vi "presention_showoff.vi"() -> ()   [LabVIEW 2012]
uses:
  <vilib>/NXT/Subs/LVHSConnector.ctl
  <vilib>/NXT/Subs/MotorOutput.ctl
  <vilib>/NXT/Block Support/NXT_InputPort.ctl
  <vilib>/NXT/Dual Mode Library/Motors/MotorOn.vi
  <vilib>/NXT/Dual Mode Library/Motors/MotorReverse.vi
  <vilib>/NXT/Dual Mode Library/Motors/MotorBrake.vi
  <vilib>/NXT/Dual Mode Library/Display/clearDisplay.vi
  <vilib>/NXT/Dual Mode Library/Waits/Wait_Num(msec).vi
  <vilib>/NXT/Dual Mode Library/Display/drawLine.vi
  <vilib>/NXT/Dual Mode Library/Display/drawNumber.vi
  <vilib>/NXT/Dual Mode Library/Display/drawCircle.vi
  <vilib>/NXT/Dual Mode Library/Waits/Wait_Num.vi
  <vilib>/NXT/Dual Mode Library/prims/addArrayElements_int.vi
  <vilib>/NXT/Dual Mode Library/prims/rotateArray/rotateArray_int.vi
  <vilib>/NXT/Dual Mode Library/Display/drawText.vi
  <vilib>/NXT/Dual Mode Library/Sound/Tone.vi
panel:
  in  "array length 2":i32
  in  "length around index 2":i32
  in  "index 2":i32
  in  "Array 7":i16[](array[numeric])
  out "Array 6":i32[](array[numeric])
  in  "clear (T/F) 4":bool
  in  "array 5":i32[](array[numeric])
  out "NXT 14":T1={"Hardware"="NXT", "Flattened String"=""}
  in  "NXT 13":T1={"Hardware"="NXT", "Flattened String"=""}
  in  "clear (T/F) 3":bool
  in  "array 4":i32[](array[numeric])
  out "NXT 12":T1={"Hardware"="NXT", "Flattened String"=""}
  in  "NXT 11":T1={"Hardware"="NXT", "Flattened String"=""}
  in  "clear (T/F) 2":bool
  in  "array 3":i32[](array[numeric])
  out "NXT 10":T1={"Hardware"="NXT", "Flattened String"=""}
  in  "NXT 9":T1={"Hardware"="NXT", "Flattened String"=""}
  out "Array 5":i16[](array[numeric])
  in  "array 2":i16[](array[numeric])
  out "Array 4":i32[](array[numeric])
  in  "Array 3":i16[](array[numeric])
  in  "clear (T/F)":bool
  in  "array":i32[](array[numeric])
  out "NXT 8":T1={"Hardware"="NXT", "Flattened String"=""}
  in  "NXT 7":T1={"Hardware"="NXT", "Flattened String"=""}
  out "debug array":i32[](array[numeric])
  in  "Array":i16[](array[numeric])
  out "Array 2":i32[](array[numeric])
  out "stuck":bool
  out "NXT 6":T1 caption="NXT"
  in  "min distance":i32=50
  in  "power 2":i32=50
  in  "NXT 5":T1
  in  "power":u16=75
  in  "degrees to  rotate":dbl
  in  "right(T)/left(F) 2":bool
  in  "NXT 4":T1={"Hardware"="NXT", "Flattened String"=""}
  out "NXT 3":T1={"Hardware"="NXT", "Flattened String"=""}
  out "NXT 2":T1={"Hardware"="NXT", "Flattened String"=""}
  out "right(T)/left(F)":bool
  out "angle":dbl
  in  "NXT":T1={"Hardware"="NXT", "Flattened String"=""}
types:
  T1 = typedef "LVHSConnector.ctl" = cluster{"Hardware":string, "Flattened String":string}
  T2 = cluster{"Origin X":i16, "Origin Y":i16, "Radius":u8}
  T3 = typedef "MotorOutput.ctl" = u8
  T4 = typedef "NXT_InputPort.ctl" = u8
  T5 = cluster{"x-y*floor(x/y)":i32, "Start X":i16, "x-y*floor(x/y)":i32, i16}
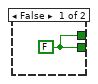
[diagram p2: hidden frame]
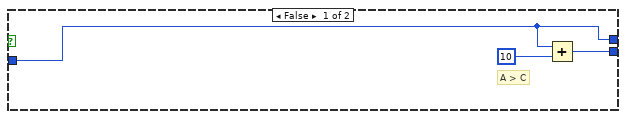
[diagram p3: hidden frame]
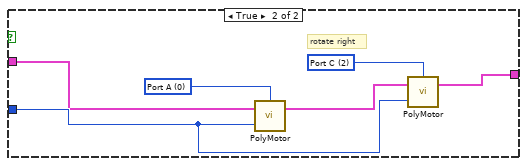
[diagram p5: hidden frame]
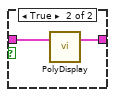
[diagram p7: hidden frame]
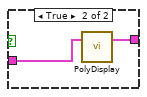
[diagram p12: hidden frame]
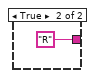
[diagram p14: hidden frame]
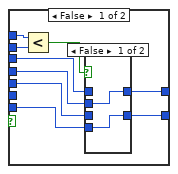
[diagram p17: hidden frame]
diagram:
  n1 = while {
    stop <- FALSE stop-if-true
    w7 = 0
    w10 = T3 5 items=["Port A"=0, "Port B"=1, "Port C"=2, "Ports A & B"=4, "Ports A & C"=5, "Ports B & C"=6, "All Ports"=3] ("Output Port (All Ports)")
    w8 = T3 5 items=["Port A"=0, "Port B"=1, "Port C"=2, "Ports A & B"=4, "Ports A & C"=5, "Ports B & C"=6, "All Ports"=3] ("Output Port (All Ports)")
    w14 = T3 5 items=["Port A"=0, "Port B"=1, "Port C"=2, "Ports A & B"=4, "Ports A & C"=5, "Ports B & C"=6, "All Ports"=3] ("Port (All Ports)")
    w22 = T3 5 items=["Port A"=0, "Port B"=1, "Port C"=2, "Ports A & B"=4, "Ports A & C"=5, "Ports B & C"=6, "All Ports"=3] ("Port (All Ports)")
    w46 = T3 5 items=["Port A"=0, "Port B"=1, "Port C"=2, "Ports A & B"=4, "Ports A & C"=5, "Ports B & C"=6, "All Ports"=3] ("Port (All Ports)")
    w52 = T3 5 items=["Port A"=0, "Port B"=1, "Port C"=2, "Ports A & B"=4, "Ports A & C"=5, "Ports B & C"=6, "All Ports"=3] ("Port (All Ports)")
    w56 = T3 2 items=["Port A"=0, "Port B"=1, "Port C"=2, "Ports A & B"=4, "Ports A & C"=5, "Ports B & C"=6, "as"=3] ("Output Port (All Ports)")
    w54 = T3 0 items=["Port A"=0, "Port B"=1, "Port C"=2, "Ports A & B"=4, "Ports A & C"=5, "Ports B & C"=6, "as"=3] ("Output Port (All Ports)")
    w69 = i16 -1 ("Start X")
    w42 = TRUE
    w51 = 35 ("Power (75)")
    w91 = T3 5 items=["Port A"=0, "Port B"=1, "Port C"=2, "Ports A & B"=4, "Ports A & C"=5, "Ports B & C"=6, "All Ports"=3] ("Port (All Ports)")
    # "Drive forward in a stright line.\nStop if:\n distance to wall is less then X.\n one of the wheels stops rotating"
    # "rotations"
    # "motor C"
    # "motor A"
    # "40"
    # "rotate left"
    # "move sensor back"
    # "if sample angle is > 180, rotate right instead of left"
    # "number of distance samples"
    # "degrees"
    # "minumum candedata size"
    # "find the closest turn candedate to the forward faceing direction with area over a given minimum\nor the largest if non over the minimum are found"
    # "msecs between distance sampling"
    # "right max"
    # "left max"
    # "area"
    # "location"
    # "debug"
    # "screen: 99x63"
    # "ResetMotor.vithe rotate vi also does this,\nbut it does not work unless also done here"
    n2 = call <vilib>:"ResetMotor.vi"("NXT"="NXT 4", "Port (All Ports)"=w14) -> ("NXT"=w12:T1)  [unwired: 2 in]
    n3 = call <vilib>:"ResetMotor.vi"("NXT"="NXT 5", "Port (All Ports)"=w8) -> ("NXT"=w9:T1)  [unwired: 2 in]
    n4 = call <vilib>:"ResetMotor.vi"("NXT"="NXT", "Port (All Ports)"=w52) -> ("NXT"=w53:T1)  [unwired: 2 in]
    n5 = call-poly <vilib>:"PolyWait.vi"("Time (100 msec)"=i16 100 ("y"), "NXT"=w12) -> ("NXT"=w11:T1)  [unwired: 2 in]
    n6 = while {
      tunnel: w9 -> [w120]
      tunnel: [w107] -> w6
      shift-right: [w101] -> _
      shift-left: w7 -> [w102]
      shift-right: [w97] -> _
      shift-left: w7 -> [w98]
      tunnel: "min distance" -> [w109]
      tunnel: "power 2" -> [w105]
      tunnel: [w92] -> w1
      stop <- w95 stop-if-true
      w113 = T3 2 items=["Port A"=0, "Port B"=1, "Port C"=2, "Ports A & B"=4, "Ports A & C"=5, "Ports B & C"=6, "All Ports"=3] ("Output Port (All Ports)")
      w114 = T3 0 items=["Port A"=0, "Port B"=1, "Port C"=2, "Ports A & B"=4, "Ports A & C"=5, "Ports B & C"=6, "All Ports"=3] ("Output Port (All Ports)")
      w115 = T3 2 items=["Port A"=0, "Port B"=1, "Port C"=2, "Ports A & B"=4, "Ports A & C"=5, "Ports B & C"=6, "All Ports"=3] ("Output Port (All Ports)")
      w116 = T3 0 items=["Port A"=0, "Port B"=1, "Port C"=2, "Ports A & B"=4, "Ports A & C"=5, "Ports B & C"=6, "All Ports"=3] ("Output Port (All Ports)")
      w121 = T4 3 items=["Port 1", "Port 2", "Port 3", "Port 4"] ("Port (Port 4)")
      n7 = call <vilib>:"Rotation.vi"("NXT"=w120, "Port (Port A)"=w114) -> ("Angle of Rotation"=w101:i32, "NXT"=w119:T1)  [unwired: 1 in]
      n8 = Equal?(x=w102, y=w101) -> (x = y?=w100:bool)
      n9 = call <vilib>:"Rotation.vi"("NXT"=w119, "Port (Port A)"=w113) -> ("Angle of Rotation"=w97:i32, "NXT"=w118:T1)  [unwired: 1 in]
      n10 = Greater?(x=w97, y=w101) -> ()  [unwired: 1 out]
      n11 = Equal?(x=w101, y=w97) -> (x = y?=w112:bool)
      n12 = Equal?(x=w98, y=w97) -> (x = y?=w99:bool)
      n13 = Or(x=w100, y=w99) -> (x .or. y?=w94:bool)
      n14 = case shown="False" w112 {
        tunnel: [w127 w136] -> w108
        tunnel: w105 -> [w128 w136]
        tunnel: [w126 w136] -> w104
        tunnel: w97 -> [w125 _]
        tunnel: w101 -> [w124 _]
        frame False {
          n15 = Greater?(x=w124, y=w125) -> (0:w129:bool)
          n16 = case shown="True" w129 {
            tunnel: w128 -> [w130 w133]
            tunnel: [w130 w134] -> w127
            tunnel: [w131 w133] -> w126
            frame False {
              # "A > C"
              n17 = Add(x=w130, y=10) -> (x+y=w131:i32)
            }
            frame True {
              # "C > A"
              n18 = Add(x=w133, y=10) -> (x+y=w134:i32)
            }
          }
        }
        frame True {
        }
      }
      n19 = case shown="True" w94 {
        tunnel: [w122 w123] -> w93
        tunnel: [w122 w123] -> w92
        frame False {
          w122 = FALSE
        }
        frame True {
          w123 = FALSE
        }
      }
      n20 = call <vilib>:"Sonar_cm.vi"("NXT"=w118, "Port (Port 4)"=w121) -> ("Distance (cm)"=w110:i16, "NXT"=w111:T1)  [unwired: 1 in]
      n21 = Less Or Equal?(x=w110, y=w109) -> (x <= y?=w96:bool)
      n22 = Or(x=w93, y=w96) -> (x .or. y?=w95:bool)
      n23 = call-poly <vilib>:"PolyMotor.vi"("Power (75)"=w108, "NXT"=w111, "Output Port (All Ports)"=w116) -> ("NXT"=w117:T1)  [unwired: 1 in]
      n24 = call-poly <vilib>:"PolyMotor.vi"("Power (75)"=w104, "NXT"=w117, "Output Port (All Ports)"=w115) -> ("NXT"=w103:T1)  [unwired: 1 in]
      n25 = call-poly <vilib>:"PolyWait.vi"("Time (100 msec)"=100, "NXT"=w103) -> ("NXT"=w107:T1)  [unwired: 2 in]
    }
    "stuck" <- w1
    n26 = call-poly <vilib>:"PolyMotor.vi"("Power (75)"=w51, "NXT"=w53, "Output Port (All Ports)"=w54) -> ("NXT"=w55:T1)  [unwired: 1 in]
    n27 = case shown="False" "right(T)/left(F) 2" {
      tunnel: "power" -> [w138 w144]
      tunnel: w11 -> [w137 w143]
      tunnel: [w139 w145] -> w25
      frame False {
        w142 = T3 2 items=["Port A"=0, "Port B"=1, "Port C"=2, "Ports A & B"=4, "Ports A & C"=5, "Ports B & C"=6, "as"=3] ("Output Port (All Ports)")
        w140 = T3 0 items=["Port A"=0, "Port B"=1, "Port C"=2, "Ports A & B"=4, "Ports A & C"=5, "Ports B & C"=6, "as"=3] ("Output Port (All Ports)")
        # "rotate left"
        n28 = call-poly <vilib>:"PolyMotor.vi"("Power (75)"=w138, "NXT"=w137, "Output Port (All Ports)"=w140) -> ("NXT"=w141:T1)  [unwired: 1 in]
        n29 = call-poly <vilib>:"PolyMotor.vi"("Power (75)"=w138, "NXT"=w141, "Output Port (All Ports)"=w142) -> ("NXT"=w139:T1)  [unwired: 1 in]
      }
      frame True {
        w148 = T3 2 items=["Port A"=0, "Port B"=1, "Port C"=2, "Ports A & B"=4, "Ports A & C"=5, "Ports B & C"=6, "as"=3] ("Output Port (All Ports)")
        w146 = T3 0 items=["Port A"=0, "Port B"=1, "Port C"=2, "Ports A & B"=4, "Ports A & C"=5, "Ports B & C"=6, "as"=3] ("Output Port (All Ports)")
        # "rotate right"
        n30 = call-poly <vilib>:"PolyMotor.vi"("Power (75)"=w144, "NXT"=w143, "Output Port (All Ports)"=w146) -> ("NXT"=w147:T1)  [unwired: 1 in]
        n31 = call-poly <vilib>:"PolyMotor.vi"("Power (75)"=w144, "NXT"=w147, "Output Port (All Ports)"=w148) -> ("NXT"=w145:T1)  [unwired: 1 in]
      }
    }
    n32 = call-poly <vilib>:"PolyMotor.vi"("Power (75)"=w51, "NXT"=w55, "Output Port (All Ports)"=w56) -> ("NXT"=w50:T1)  [unwired: 1 in]
    n33 = Multiply(x=360.0 ("Max Value"), y=1.45 ("Max Value")) -> (x*y=w47:dbl)
    n34 = while {
      shift-right: [w253] -> w30
      shift-left: i16[] [] -> [w254]
      tunnel: [w250] -> w45
      tunnel: w42 -> [w249]
      tunnel: 7 -> [w246]
      tunnel: w50 -> [w235]
      tunnel: w47 -> [w232]
      i -> [w247]
      stop <- w233 stop-if-true
      w243 = T3 2 items=["Port A"=0, "Port B"=1, "Port C"=2, "Ports A & B"=4, "Ports A & C"=5, "Ports B & C"=6, "as"=3] ("Output Port (All Ports)")
      w244 = T3 0 items=["Port A"=0, "Port B"=1, "Port C"=2, "Ports A & B"=4, "Ports A & C"=5, "Ports B & C"=6, "as"=3] ("Output Port (All Ports)")
      w255 = T4 3 items=["Port 1", "Port 2", "Port 3", "Port 4"] ("Port (Port 4)")
      n35 = call <vilib>:"Rotation.vi"("NXT"=w235, "Port (Port A)"=w244) -> ("Angle of Rotation"=w242:i32, "NXT"=w245:T1)  [unwired: 1 in]
      n36 = call <vilib>:"Rotation.vi"("NXT"=w245, "Port (Port A)"=w243) -> ("Angle of Rotation"=w241:i32, "NXT"=w234:T1)  [unwired: 1 in]
      n37 = Absolute Value(x=w241) -> (abs(x)=w239:i32)
      n38 = Absolute Value(x=w242) -> (abs(x)=w240:i32)
      n39 = Add(x=w239, y=w240) -> (x+y=w238:i32)
      n40 = call <vilib>:"Sonar_cm.vi"("NXT"=w234, "Port (Port 4)"=w255) -> ("Distance (cm)"=w248:i16, "NXT"=w252:T1)  [unwired: 1 in]
      n41 = call-poly <vilib>:"PolyWait.vi"("Time (100 msec)"=w246, "NXT"=w252) -> ("NXT"=w251:T1)  [unwired: 2 in]
      n42 = Divide(x=w238, y=2) -> (x/y=w236:dbl)
      n43 = Greater Or Equal?(x=w236, y=w232) -> (x >= y?=w233:bool)
      n44 = case shown="True" w249 {
        tunnel: w251 -> [w256 w266]
        tunnel: [w256 w267] -> w250
        tunnel: w248 -> [_ w265]
        tunnel: w247 -> [_ w258]
        frame False {
        }
        frame True {
          n45 = Divide(x=i16 60 ("Start X"), y=i16 255 ("Start X")) -> (x/y=w263:dbl)
          n46 = Multiply(x=w265, y=w263) -> (x*y=w268:dbl)
          n47 = call <vilib>:"quot_Remain.vi"("y"=i16 99 ("Start X"), "x"=w258) -> ("x-y*floor(x/y)"=w259:i32)  [unwired: 1 out]
          n48 = To Word Integer(number=w268) -> (16bit integer=w260:i16)
          n49 = Bundle("x-y*floor(x/y)"=w259, "Start X"=i16 0, "x-y*floor(x/y)"=w259, w260) -> (w261:T5)  [unwired: 1 in]
          n50 = call-poly <vilib>:"PolyDisplay.vi"("Line Parameters"=w261, "NXT"=w266) -> ("NXT"=w267:T1)  [unwired: 2 in]
        }
      }
      n51 = Build Array (concatenate)(w254, w248) -> (w253:i16[])
    }
    n52 = Multiply(x="degrees to  rotate", y=1.475 ("Max Value")) -> (x*y=w21:dbl)
    n53 = while {
      tunnel: w25 -> [w162]
      tunnel: w21 -> [w152]
      tunnel: [w149] -> w23
      stop <- w150 stop-if-true
      w159 = T3 2 items=["Port A"=0, "Port B"=1, "Port C"=2, "Ports A & B"=4, "Ports A & C"=5, "Ports B & C"=6, "as"=3] ("Output Port (All Ports)")
      w160 = T3 0 items=["Port A"=0, "Port B"=1, "Port C"=2, "Ports A & B"=4, "Ports A & C"=5, "Ports B & C"=6, "as"=3] ("Output Port (All Ports)")
      n54 = call <vilib>:"Rotation.vi"("NXT"=w162, "Port (Port A)"=w160) -> ("Angle of Rotation"=w158:i32, "NXT"=w161:T1)  [unwired: 1 in]
      n55 = call <vilib>:"Rotation.vi"("NXT"=w161, "Port (Port A)"=w159) -> ("Angle of Rotation"=w157:i32, "NXT"=w149:T1)  [unwired: 1 in]
      n56 = Absolute Value(x=w157) -> (abs(x)=w155:i32)
      n57 = Absolute Value(x=w158) -> (abs(x)=w156:i32)
      n58 = Add(x=w155, y=w156) -> (x+y=w154:i32)
      n59 = Divide(x=w154, y=2) -> (x/y=w151:dbl)
      n60 = Greater Or Equal?(x=w151, y=w152) -> (x >= y?=w150:bool)
    }
    n61 = call-poly <vilib>:"PolyMotor.vi"("NXT"=w23, "Port (All Ports)"=w22) -> ("NXT"=w17:T1)  [unwired: 2 in]
    n62 = call-poly <vilib>:"PolyWait.vi"("Time (100 msec)"=i16 100 ("y"), "NXT"=w17) -> ("NXT"=→"NXT 3":T1)  [unwired: 2 in]
    n63 = call-poly <vilib>:"PolyMotor.vi"("NXT"=w6, "Port (All Ports)"=w10) -> ("NXT"=→"NXT 6":T1)  [unwired: 2 in]
    n64 = call-poly <vilib>:"PolyMotor.vi"("NXT"=w45, "Port (All Ports)"=w46) -> ("NXT"=w44:T1)  [unwired: 2 in]
    n65 = case shown="True" w42 {
      tunnel: w44 -> [w163 w189]
      tunnel: [w163 w182] -> w43
      tunnel: w30 -> [_ w187]
      frame False {
      }
      frame True {
        w168 = i16 0 items=["1", "2", "3", "4", "5", "6", "7", "8"] ("Line")
        w171 = i16 7 items=["1", "2", "3", "4", "5", "6", "7", "8"] ("Line")
        (unwired) i16 255 ("Start X")
        # "max value"
        # "fit raw data to screen"
        # "pause while displaying raw data"
        n66 = while {
          tunnel: w189 -> [w230]
          tunnel: [w229] -> w185
          stop <- w231 stop-if-true
          n67 = call <vilib>:"readNXTButton.vi"("NXT"=w230) -> ("Yes/No"=w231:bool, "NXT"=w229:T1)  [unwired: 2 in]
        }
        n68 = for {
          tunnel: "array" -> [w195] mode=indexing
          tunnel: "array" -> [w197]
          tunnel: [w197] -> w176
          shift-right: [w194] -> w170
          shift-left: i16 -1 ("Start X") -> [w193]
          n69 = Greater?(x=w195, y=w193) -> (0:w196:bool)
          n70 = case shown="True" w196 {
            tunnel: w195 -> [_ w199]
            tunnel: [w198 w199] -> w194
            tunnel: w193 -> [w198 _]
            frame False {
            }
            frame True {
            }
          }
        }
        n71 = case shown="False" "clear (T/F)" {
          tunnel: "NXT 7" -> [w190 w192]
          tunnel: [w190 w191] -> w167
          frame False {
          }
          frame True {
            n72 = call-poly <vilib>:"PolyDisplay.vi"("NXT"=w192) -> ("NXT"=w191:T1)  [unwired: 3 in]
          }
        }
        n73 = Array Size(array=w176) -> (size(s)=w166:i32)
        n74 = Divide(x=i16 30 ("Start X"), y=w170) -> (x/y=w180:dbl)
        n75 = call-poly <vilib>:"PolyDisplay.vi"("number"=w166, "NXT"=w167, "Line"=w168) -> ("NXT"=w165:T1)  [unwired: 1 in]
        n76 = call-poly <vilib>:"PolyDisplay.vi"("number"=w170, "NXT"=w165, "Line"=w171) -> ("NXT"=w172:T1)  [unwired: 1 in]
        n77 = call-poly <vilib>:"PolyDisplay.vi"("Circle Parameters"=T2 {"Origin X"=49, "Origin Y"=31, "Radius"=30}, "NXT"=w172) -> ("NXT"=w173:T1)  [unwired: 2 in]
        n78 = for {
          N: w166 -> [_]
          tunnel: [w219] -> w178
          tunnel: w180 -> [w223]
          tunnel: w173 -> [w222]
          tunnel: w176 -> [w221]
          tunnel: w166 -> [w204]
          i -> [w205]
          w213 = i16 49 ("Start X")
          w211 = i16 31 ("Start X")
          # "shift"
          # "dx"
          # "dy"
          # "radians"
          # "magnitude"
          n79 = Index Array(array=w221, index=w205) -> (element=w220:i32)
          n80 = Divide(x=w205, y=w204) -> (x/y=w218:dbl)
          n81 = Multiply(x=w220, y=w223) -> (x*y=w212:dbl)
          n82 = Multiply(x=w218, y=6.283185307179586 ("Pi Multiplied By 2")) -> (x*y=w202:dbl)
          n83 = Add(x=w202, y=1.5707963267948966 ("Pi Divided By 2")) -> (x+y=w201:dbl)
          n84 = call <vilib>:"cosine.vi"("x"=w201) -> ("cos(x)"=w215:sgl)
          n85 = call <vilib>:"sine.vi"("x"=w201) -> ("sin(x)"=w216:sgl)
          n86 = Multiply(x=w215, y=w212) -> (x*y=w214:dbl)
          n87 = Multiply(x=w216, y=w212) -> (x*y=w203:dbl)
          n88 = Add(x=w214, y=w213) -> (x+y=w209:dbl)
          n89 = Add(x=w211, y=w203) -> (x+y=w207:dbl)
          n90 = To Word Integer(number=w209) -> (16bit integer=w208:i16)
          n91 = To Word Integer(number=w207) -> (16bit integer=w206:i16)
          n92 = Bundle("Start X"=w213, "Start X"=w211, w208, w206) -> (w210:cluster{"Start X":i16, "Start X":i16, i16, i16})  [unwired: 1 in]
          n93 = call-poly <vilib>:"PolyDisplay.vi"("Line Parameters"=w210, "NXT"=w222) -> ("NXT"=w219:T1)  [unwired: 2 in]
        }
        "NXT 8" <- w178
        n94 = call-poly <vilib>:"PolyWait.vi"("Time (1 sec)"=i16 1, "NXT"=w185) -> ("NXT"=w184:T1)  [unwired: 2 in]
        n95 = call "radial_array_display.vi"("array"=w187, "clear (T/F)"=TRUE, "NXT"=w184) -> ("NXT 2"=w188:T1)  [unwired: 8 in]
        n96 = while {
          tunnel: w188 -> [w227]
          tunnel: [w226] -> w181
          stop <- w228 stop-if-true
          n97 = call <vilib>:"readNXTButton.vi"("NXT"=w227) -> ("Yes/No"=w228:bool, "NXT"=w226:T1)  [unwired: 2 in]
        }
        n98 = stacked-sequence {
          tunnel: w181 -> [w225]
          tunnel: [w225] -> w182
          frame #0 {
            n99 = Wait (ms)(milliseconds to wait=u32 1000) -> ()  [unwired: 1 out]
          }
        }
      }
    }
    n100 = stacked-sequence {
      tunnel: w30 -> [w901]
      tunnel: [w899] -> w81
      tunnel: w43 -> [w900]
      tunnel: [w900] -> w40
      frame #0 {
        w885 = i16 2 ("x")
        # "ERROR IF 4\n(ONLY ON nxt)"
        # "? FILE ERROR ON nxt IF ARRAY IS INDEXED WITH A DOUBLE"
        # "guassian kernel functions:\n(expt float-e (- (* 4 n n)) => (0.237 0.698 1.0 0.698 0.237)\n(expt float-e (- (* n n)))  =>  (0.698 0.914 1.0 0.914 0.698)"
        # "start index"
        # "(defun smooth (l)\n  (let* ((kern-sum (reduce '+ kern))\n\t (len (length l))\n\t (llen (+ len 4))\n\t (list (append (subseq l (- len 2)) l (subseq l 0 2)))\n\t ;;(i 3) ;;start index (of the next element to be added to `ksub')\n\t (i 5)\n\t (ksub (subseq list 0 5)) ;;1 6)) \n\t newlist)\n\t\n    (while (<= i llen) \n      (push (/ (reduce '+ (mapcar* '* ksub kern)) kern-sum)\n\t    newlist)\n      (pop ksub)\n      (setq ksub (append ksub (list (nth i list))))\n      (setq i (1+ i)))\n    (reverse newlist)))"
        # "array length"
        n101 = call "filter_bad_values.vi"("Array 3"=w901) -> ("Array 4"=w898:i32[])  [unwired: 10 in]
        n102 = Array Size(array="array 2") -> (size(s)=w879:i32)
        n103 = Array Subset(array="Array 3", index=0, length=3 ("index")) -> (w892:i16[])
        n104 = Subtract(x=w879, y=w885) -> (x-y=w886:i32)
        n105 = Build Array (concatenate)("Array 3", w892) -> (w891:i16[])
        n106 = call "kernal_smooth.vi"("array"=w898) -> ("Array"=w899:i16[])  [unwired: 10 in]
        n107 = Add(x=i16 3, y=w879) -> (x+y=w878:i32)
        n108 = Array Size(array=w891) -> (size(s)=w896:i32)
        n109 = Array Subset(array="array 2", index=w886, length=w885) -> (w881:i16[])
        n110 = Array Subset(array="array 2", index=i16 0 ("x"), length=i16 2 ("x")) -> (w882:i16[])
        n111 = Build Array (concatenate)(w882, "array 2", w881) -> (w867:i16[])
        n112 = Subtract(x=w896, y=3) -> (x-y=w889:i32)
        n113 = Index Array(array=w867, index=i16 0 ("x")) -> (element=w877:i16)
        n114 = Index Array(array=w867, index=i16 4 ("x")) -> (element=w869:i16)
        n115 = Index Array(array=w867, index=i16 1 ("x")) -> (element=w872:i16)
        n116 = Index Array(array=w867, index=i16 3 ("x")) -> (element=w870:i16)
        n117 = Index Array(array=w867, index=i16 2 ("x")) -> (element=w871:i16)
        n118 = for {
          N: w889 -> [_]
          tunnel: w891 -> [w932]
          shift-right: [w933] -> w888
          shift-left: i32[] [] -> [w934]
          tunnel: w889 -> [w937]
          tunnel: "Array 3" -> [w931]
          i -> [w938]
          w939 = 255
          w946 = 1
          n119 = Index Array(array=w932, index=w938) -> (element=w936:i16)
          n120 = Add(x=w938, y=w946) -> (x+y=w945:i32)
          n121 = Equal?(x=w939, y=w936) -> (x = y?=w943:bool)
          n122 = Index Array(array=w932, index=w945) -> (element=w942:i16)
          n123 = Add(x=w945, y=w946) -> (x+y=w944:i32)
          n124 = Add(x=w944, y=w946) -> (x+y=w947:i32)
          n125 = Index Array(array=w932, index=w944) -> (element=w941:i16)
          n126 = Index Array(array=w932, index=w947) -> (element=w940:i16)
          n127 = case shown="True" w943 {
            tunnel: w942 -> [_ w959]
            tunnel: w941 -> [_ w960]
            tunnel: w940 -> [_ w961]
            tunnel: w939 -> [_ w953]
            tunnel: w938 -> [_ w952]
            tunnel: w937 -> [_ w951]
            tunnel: [w948 w950] -> w935
            tunnel: w936 -> [w948 _]
            tunnel: w931 -> [_ w949]
            frame False {
            }
            frame True {
              n128 = Equal?(x=w953, y=w959) -> (x = y?=w958:bool)
              n129 = Equal?(x=w953, y=w960) -> (x = y?=w957:bool)
              n130 = Equal?(x=w953, y=w961) -> (x = y?=w955:bool)
              n131 = And(x=w958, y=w957) -> (x .and. y?=w956:bool)
              n132 = And(x=w956, y=w955) -> (x .and. y?=w954:bool)
              n133 = case shown="False" w954 {
                tunnel: w953 -> [_ w1023]
                tunnel: [w982 w1023] -> w950
                tunnel: w952 -> [w989 _]
                tunnel: w951 -> [w988 _]
                tunnel: w949 -> [w979 _]
                frame False {
                  # "len around ind."
                  # "array"
                  # "index"
                  # "return a new array of values around an index in an array treated as a ring"
                  # "average surounding values != 255"
                  n134 = call "subseq_around_index.vi"("length around index 2"=3 ("length around index"), "index 2"=w989, "array length 2"=w988, "Array 3"=w979) -> ("Array 2"=w987:i32[])  [unwired: 7 in]
                  n135 = Subtract(x="array length 2", y="length around index 2") -> (x-y=w976:i32)
                  n136 = Less?(x="index 2", y="length around index 2") -> (x < y?=w978:bool)
                  n137 = Greater Or Equal?(x="index 2", y=w976) -> (x >= y?=w975:bool)
                  n138 = Or(x=w975, y=w978) -> (x .or. y?=w977:bool)
                  n139 = for {
                    tunnel: w987 -> [w1016] mode=indexing
                    shift-right: [w1015] -> w984
                    shift-left: i32[] [] -> [w1014]
                    n140 = Not Equal?(x=255 ("y"), y=w1016) -> (x != y?=w1018:bool)
                    n141 = case shown="True" w1018 {
                      tunnel: w1016 -> [_ w1022]
                      tunnel: [w1019 w1021] -> w1015
                      tunnel: w1014 -> [w1019 w1020]
                      frame False {
                      }
                      frame True {
                        n142 = Build Array (concatenate)(w1020, w1022) -> (w1021:i32[])
                      }
                    }
                  }
                  n143 = case shown="True" w977 {
                    tunnel: w975 -> [_ w999]
                    tunnel: "array length 2" -> [_ w996]
                    tunnel: "length around index 2" -> [w991 w993]
                    tunnel: "Array 7" -> [w992 w998]
                    tunnel: "index 2" -> [w990 w997]
                    tunnel: [w992 w994] -> w972
                    tunnel: [w991 w993] -> w971
                    tunnel: [w990 w995] -> w970
                    frame False {
                      # "in middle of array"
                    }
                    frame True {
                      n144 = case shown="True" w999 {
                        tunnel: w998 -> [w1002 w1010]
                        tunnel: w997 -> [w1004 w1009]
                        tunnel: w996 -> [_ w1013]
                        tunnel: [w1001 w1007] -> w995
                        tunnel: w993 -> [w1005 _]
                        tunnel: [w1000 w1006] -> w994
                        frame False {
                          # "index"
                          # "at beginning of array"
                          n145 = Subtract(x=w1005, y=w1004) -> (x-y=w1003:i32)
                          n146 = Add(x=w1004, y=w1003) -> (x+y=w1001:i32)
                          n147 = call-poly <vilib>:"rotateArray_poly.vi"("Array"=w1002, "n"=w1003) -> ("rotated array"=w1000:i32[])
                        }
                        frame True {
                          # "index"
                          # "at end of array"
                          n148 = Subtract(x=w1013, y=w1009) -> (x-y=w1008:i32)
                          n149 = Subtract(x=w1009, y=w1008) -> (x-y=w1007:i32)
                          n150 = Multiply(x=w1008, y=-1.0) -> (x*y=w1011:dbl)
                          n151 = call-poly <vilib>:"rotateArray_poly.vi"("Array"=w1010, "n"=w1011) -> ("rotated array"=w1006:i32[])
                        }
                      }
                    }
                  }
                  n152 = Subtract(x=w970, y=w971) -> (x-y=w973:i32)
                  n153 = Add(x=1, y=w970) -> (x+y=w969:i32)
                  n154 = call-poly <vilib>:"addArrayElements_poly.vi"("Numeric Array"=w984) -> ("Sum"=w986:i32)
                  n155 = Array Size(array=w984) -> (size(s)=w985:i32)
                  n156 = Array Subset(array=w972, index=w973, length=w971) -> (w968:i32[])
                  n157 = Array Subset(array=w972, index=w969, length=w971) -> (w967:i32[])
                  n158 = Divide(x=w986, y=w985) -> (x/y=w983:dbl)
                  n159 = Build Array (concatenate)(w968, w967) -> (→"Array 6":i32[])
                  n160 = To Word Integer(number=w983) -> (16bit integer=w982:i16)
                }
                frame True {
                  # "255"
                }
              }
            }
          }
          n161 = Build Array (concatenate)(w934, w935) -> (w933:i32[])
        }
        "Array 4" <- w888
        n162 = while {
          shift-right: [w913] -> _
          shift-left: i16 5 ("x") -> [w902]
          tunnel: w878 -> [w930]
          shift-right: [w908] -> _
          shift-left: w877 -> [w929]
          shift-right: [w909] -> _
          shift-left: w872 -> [w908]
          shift-right: [w910] -> _
          shift-left: w871 -> [w909]
          shift-right: [w911] -> _
          shift-left: w870 -> [w910]
          shift-right: [w912] -> _
          shift-left: w869 -> [w911]
          tunnel: w867 -> [w924]
          shift-right: [w906] -> w865
          shift-left: i16[] [] -> [w907]
          stop <- w903 continue-if-true
          (unwired) 2.87
          # "kernal sum"
          n163 = Less?(x=w902, y=w930) -> (x < y?=w903:bool)
          n164 = Index Array(array=w924, index=w902) -> (element=w912:i16)
          n165 = Add(x=w902, y=i16 1 ("x")) -> (x+y=w913:i16)
          n166 = Multiply(x=w929, y=0.698) -> (x*y=w922:dbl)
          n167 = Multiply(x=w908, y=0.914) -> (x*y=w923:dbl)
          n168 = Multiply(x=w910, y=0.914) -> (x*y=w919:dbl)
          n169 = Multiply(x=w911, y=0.698) -> (x*y=w917:dbl)
          n170 = Add(x=w922, y=w923) -> (x+y=w921:dbl)
          n171 = Add(x=w921, y=w909) -> (x+y=w920:dbl)
          n172 = Add(x=w920, y=w919) -> (x+y=w918:dbl)
          n173 = Add(x=w918, y=w917) -> (x+y=w916:dbl)
          n174 = Divide(x=w916, y=4.22) -> (x/y=w904:dbl)
          n175 = To Word Integer(number=w904) -> (16bit integer=w905:i16)
          n176 = Build Array (concatenate)(w907, w905) -> (w906:i16[])
        }
        "Array 5" <- w865
      }
    }
    n177 = case shown="True" w42 {
      tunnel: w40 -> [w1025 w1043]
      tunnel: w81 -> [w1024 w1048]
      tunnel: [w1025 w1044] -> w78
      tunnel: [w1024 w1048] -> w80
      frame False {
      }
      frame True {
        w1030 = i16 0 items=["1", "2", "3", "4", "5", "6", "7", "8"] ("Line")
        w1033 = i16 7 items=["1", "2", "3", "4", "5", "6", "7", "8"] ("Line")
        (unwired) i16 255 ("Start X")
        # "max value"
        # "displaying filtered and smoothed data"
        # "filter and display array"
        n178 = call "radial_array_display.vi"("array"=w1048, "NXT"=w1043) -> ("NXT 2"=w1047:T1)  [unwired: 9 in]
        n179 = while {
          tunnel: w1047 -> [w1084]
          tunnel: [w1083] -> w1045
          stop <- w1085 stop-if-true
          n180 = call <vilib>:"readNXTButton.vi"("NXT"=w1084) -> ("Yes/No"=w1085:bool, "NXT"=w1083:T1)  [unwired: 2 in]
        }
        n181 = case shown="False" "clear (T/F) 2" {
          tunnel: "NXT 9" -> [w1049 w1051]
          tunnel: [w1049 w1050] -> w1029
          frame False {
          }
          frame True {
            n182 = call-poly <vilib>:"PolyDisplay.vi"("NXT"=w1051) -> ("NXT"=w1050:T1)  [unwired: 3 in]
          }
        }
        n183 = for {
          tunnel: "array 3" -> [w1054] mode=indexing
          tunnel: "array 3" -> [w1056]
          tunnel: [w1056] -> w1038
          shift-right: [w1053] -> w1032
          shift-left: i16 -1 ("Start X") -> [w1052]
          n184 = Greater?(x=w1054, y=w1052) -> (0:w1055:bool)
          n185 = case shown="True" w1055 {
            tunnel: w1054 -> [_ w1058]
            tunnel: [w1057 w1058] -> w1053
            tunnel: w1052 -> [w1057 _]
            frame False {
            }
            frame True {
            }
          }
        }
        n186 = call-poly <vilib>:"PolyWait.vi"("Time (1 sec)"=i16 1, "NXT"=w1045) -> ("NXT"=w1044:T1)  [unwired: 2 in]
        n187 = Array Size(array=w1038) -> (size(s)=w1028:i32)
        n188 = Divide(x=i16 30 ("Start X"), y=w1032) -> (x/y=w1042:dbl)
        n189 = call-poly <vilib>:"PolyDisplay.vi"("number"=w1028, "NXT"=w1029, "Line"=w1030) -> ("NXT"=w1027:T1)  [unwired: 1 in]
        n190 = call-poly <vilib>:"PolyDisplay.vi"("number"=w1032, "NXT"=w1027, "Line"=w1033) -> ("NXT"=w1034:T1)  [unwired: 1 in]
        n191 = call-poly <vilib>:"PolyDisplay.vi"("Circle Parameters"=T2 {"Origin X"=49, "Origin Y"=31, "Radius"=30}, "NXT"=w1034) -> ("NXT"=w1035:T1)  [unwired: 2 in]
        n192 = for {
          N: w1028 -> [_]
          tunnel: [w1078] -> w1040
          tunnel: w1042 -> [w1082]
          tunnel: w1035 -> [w1081]
          tunnel: w1038 -> [w1080]
          tunnel: w1028 -> [w1063]
          i -> [w1064]
          w1072 = i16 49 ("Start X")
          w1070 = i16 31 ("Start X")
          # "shift"
          # "dx"
          # "dy"
          # "radians"
          # "magnitude"
          n193 = Index Array(array=w1080, index=w1064) -> (element=w1079:i32)
          n194 = Divide(x=w1064, y=w1063) -> (x/y=w1077:dbl)
          n195 = Multiply(x=w1079, y=w1082) -> (x*y=w1071:dbl)
          n196 = Multiply(x=w1077, y=6.283185307179586 ("Pi Multiplied By 2")) -> (x*y=w1061:dbl)
          n197 = Add(x=w1061, y=1.5707963267948966 ("Pi Divided By 2")) -> (x+y=w1060:dbl)
          n198 = call <vilib>:"cosine.vi"("x"=w1060) -> ("cos(x)"=w1074:sgl)
          n199 = call <vilib>:"sine.vi"("x"=w1060) -> ("sin(x)"=w1075:sgl)
          n200 = Multiply(x=w1074, y=w1071) -> (x*y=w1073:dbl)
          n201 = Multiply(x=w1075, y=w1071) -> (x*y=w1062:dbl)
          n202 = Add(x=w1073, y=w1072) -> (x+y=w1068:dbl)
          n203 = Add(x=w1070, y=w1062) -> (x+y=w1066:dbl)
          n204 = To Word Integer(number=w1068) -> (16bit integer=w1067:i16)
          n205 = To Word Integer(number=w1066) -> (16bit integer=w1065:i16)
          n206 = Bundle("Start X"=w1072, "Start X"=w1070, w1067, w1065) -> (w1069:cluster{"Start X":i16, "Start X":i16, i16, i16})  [unwired: 1 in]
          n207 = call-poly <vilib>:"PolyDisplay.vi"("Line Parameters"=w1069, "NXT"=w1081) -> ("NXT"=w1078:T1)  [unwired: 2 in]
        }
        "NXT 10" <- w1040
      }
    }
    n208 = call-poly <vilib>:"PolyDisplay.vi"("NXT"=w78) -> ("NXT"=w61:T1)  [unwired: 3 in]
    n209 = stacked-sequence {
      tunnel: w80 -> [w514]
      tunnel: [w513] -> w79
      tunnel: [w512] -> w57
      tunnel: w61 -> [w511]
      tunnel: [w511] -> w60
      frame #0 {
        w474 = FALSE
        w473 = -1 ("x")
        w506 = 2 ("x")
        # "50 too far"
        # "?\nkeep track of \nfirst, last, area\nof the first and\nlast groups (with\nindexes starting\nat 0 or ending at\nthe array max"
        # "dont forget about the last one"
        # "60"
        # "TODO: seporate this as a vi"
        # "position--area  arrau"
        # "start--end--area  array"
        # "combine first and last candedates, if any"
        # "construct position--area array"
        # "start"
        # "in block ?"
        # "area"
        # "next index"
        # "index"
        # "min distance"
        # "found blocks"
        n210 = call "find_path.vi"("Array"=w514) -> ("debug array"=w513:i32[], "Array 2"=w512:i32[])  [unwired: 9 in]
        n211 = Array Size(array="Array") -> (size(s)=w476:i32)
        n212 = Subtract(x=w476, y=w506) -> (x-y=w507:i32)
        n213 = Subtract(x=w476, y=2 ("x")) -> (x-y=w509:i32)
        n214 = Subtract(x=w476, y=1) -> (x-y=w457:i32)
        n215 = Array Subset(array="Array", index=w507, length=w506) -> (w503:i16[])
        n216 = Array Subset(array="Array", index=0 ("x"), length=2 ("x")) -> (w508:i16[])
        n217 = Build Array (concatenate)(w508, "Array", w503) -> (w496:i16[])
        n218 = Index Array(array=w496, index=1 ("x")) -> (element=w499:i16)
        n219 = Index Array(array=w496, index=3 ("x")) -> (element=w497:i16)
        n220 = Index Array(array=w496, index=2 ("x")) -> (element=w498:i16)
        n221 = for {
          N: w509 -> [_]
          shift-right: [w687] -> _
          shift-left: w499 -> [w710]
          shift-right: [w686] -> _
          shift-left: w498 -> [w687]
          shift-right: [w706] -> _
          shift-left: w497 -> [w686]
          tunnel: w496 -> [w707]
          shift-right: [w705] -> _
          shift-left: 3 ("x") -> [w704]
          tunnel: 40 ("x") -> [w700]
          shift-right: [w696] -> w489
          shift-left: FALSE -> [w699]
          shift-right: [w697] -> w486
          shift-left: 0 ("x") -> [w698]
          shift-right: [w693] -> w488
          shift-left: 0 ("x") -> [w695]
          shift-right: [w690] -> w487
          shift-left: 0 ("x") -> [w694]
          shift-right: [w688] -> w485
          shift-left: i16[] [] -> [w692]
          # "seporate array of distance values into blocks of continuous distances"
          # "average"
          # "c"
          # "b"
          # "a"
          n222 = Add(x=w710, y=w687) -> (x+y=w711:i16)
          n223 = Index Array(array=w707, index=w704) -> (element=w706:i16)
          n224 = Add(x=w704, y=1 ("x")) -> (x+y=w705:i32)
          n225 = Add(x=w711, y=w686) -> (x+y=w709:i16)
          n226 = Divide(x=w709, y=3 ("x")) -> (x/y=w701:dbl)
          n227 = Greater?(x=w701, y=w700) -> (0:w702:bool)
          n228 = case shown="True" w702 {
            tunnel: w699 -> [w721 w742]
            tunnel: w698 -> [w716 w745]
            tunnel: w686 -> [_ w744]
            tunnel: [w715 w743] -> w697
            tunnel: [w720 w741] -> w696
            tunnel: w695 -> [w718 w740]
            tunnel: w694 -> [w717 w739]
            tunnel: [w713 w738] -> w693
            tunnel: w692 -> [w719 w736]
            tunnel: [w714 w737] -> w691
            tunnel: [w712 w735] -> w688
            frame False {
              n229 = case shown="False" w721 {
                selector: w721 -> [w724 _]
                tunnel: [w724 FALSE] -> w720
                tunnel: w719 -> [w726 w733]
                tunnel: w718 -> [w722 w728]
                tunnel: w717 -> [w723 w729]
                tunnel: w716 -> [w725 w730]
                tunnel: [w725 w730] -> w715
                tunnel: [w723 w729] -> w714
                tunnel: [w722 w728] -> w713
                tunnel: [w726 w727] -> w712
                frame False {
                }
                frame True {
                  # "area"
                  # "end"
                  # "start"
                  # "end of block"
                  n230 = Build Array (concatenate)(w733, w728) -> (w732:i32[])
                  n231 = Build Array (concatenate)(w732, w729) -> (w731:i32[])
                  n232 = Build Array (concatenate)(w731, w730) -> (w727:i32[])
                }
              }
            }
            frame True {
              n233 = case shown="True" w742 {
                tunnel: w745 -> [_ w756]
                tunnel: w744 -> [w746 w755]
                tunnel: [w746 w754] -> w743
                tunnel: w742 -> [_ w753]
                tunnel: [TRUE w753] -> w741
                tunnel: w740 -> [_ w752]
                tunnel: w739 -> [w748 w751]
                tunnel: [w748 w752] -> w738
                tunnel: [w748 w751] -> w737
                tunnel: w736 -> [w747 w750]
                tunnel: [w747 w750] -> w735
                frame False {
                  # "block start"
                }
                frame True {
                  # "in block"
                  n234 = Add(x=w755, y=w756) -> (x+y=w754:i32)
                }
              }
            }
          }
          n235 = Add(x=w691, y=1 ("x")) -> (x+y=w690:i32)
        }
        n236 = case shown="True" w489 {
          tunnel: w488 -> [_ w683]
          tunnel: w487 -> [_ w680]
          tunnel: w486 -> [_ w679]
          tunnel: [w676 w678] -> w445
          tunnel: w485 -> [w676 w677]
          frame False {
          }
          frame True {
            # "area"
            # "end"
            # "start"
            n237 = Build Array (concatenate)(w677, w683) -> (w684:i32[])
            n238 = Add(x=w680, y=1 ("x")) -> (x+y=w681:i32)
            n239 = Build Array (concatenate)(w684, w681) -> (w685:i32[])
            n240 = Build Array (concatenate)(w685, w679) -> (w678:i32[])
          }
        }
        "debug array" <- w445
        n241 = Array Size(array=w445) -> (size(s)=w483:i32)
        n242 = Divide(x=w483, y=3) -> (x/y=w481:dbl)
        n243 = To Word Integer(number=w481) -> (16bit integer=w480:i16)
        n244 = for {
          N: w480 -> [_]
          tunnel: w445 -> [w605]
          shift-right: [w586] -> w460
          shift-left: w473 -> [w598]
          shift-right: [w585] -> w461
          shift-left: w473 -> [w597]
          shift-right: [w584] -> w462
          shift-left: w473 -> [w596]
          shift-right: [w591] -> w463
          shift-left: w473 -> [w595]
          shift-right: [w589] -> w464
          shift-left: w473 -> [w594]
          shift-right: [w587] -> w465
          shift-left: w473 -> [w593]
          shift-right: [w606] -> _
          shift-left: 0 ("x") -> [w592]
          shift-right: [w607] -> _
          shift-left: 1 ("x") -> [w590]
          shift-right: [w608] -> _
          shift-left: 2 ("x") -> [w588]
          tunnel: w457 -> [w599]
          shift-right: [w580] -> w469
          shift-left: w474 -> [w582]
          shift-right: [w581] -> w470
          shift-left: w474 -> [w583]
          shift-right: [w578] -> w459
          shift-left: i16[] [] -> [w579]
          tunnel: "Array" -> [w574]
          tunnel: TRUE -> [w573]
          w604 = 3 ("x")
          n245 = Index Array(array=w605, index=w590) -> (element=w576:i32)
          n246 = Index Array(array=w605, index=w592) -> (element=w575:i32)
          n247 = Index Array(array=w605, index=w588) -> (element=w577:i32)
          n248 = Add(x=w588, y=w604) -> (x+y=w608:i32)
          n249 = Equal?(x=w576, y=w599) -> (x = y?=w603:bool)
          n250 = Add(x=w604, y=w592) -> (x+y=w606:i32)
          n251 = Add(x=w604, y=w590) -> (x+y=w607:i32)
          n252 = Equal?(x=w575, y=0 ("x")) -> (x = y?=w600:bool)
          n253 = Or(x=w600, y=w603) -> (x .or. y?=w602:bool)
          n254 = case shown="False" w602 {
            tunnel: w600 -> [_ w657]
            tunnel: w598 -> [w625 w656]
            tunnel: w597 -> [w624 w655]
            tunnel: w596 -> [w623 w654]
            tunnel: w595 -> [w622 w653]
            tunnel: w594 -> [w621 w652]
            tunnel: w593 -> [w620 w651]
            tunnel: w575 -> [w614 w650]
            tunnel: [w622 w649] -> w591
            tunnel: w576 -> [w615 w648]
            tunnel: [w621 w647] -> w589
            tunnel: w577 -> [w617 w646]
            tunnel: [w620 w645] -> w587
            tunnel: [w625 w644] -> w586
            tunnel: [w624 w643] -> w585
            tunnel: [w623 w642] -> w584
            tunnel: w583 -> [w619 w641]
            tunnel: w582 -> [w618 w640]
            tunnel: [w618 w639] -> w580
            tunnel: [w619 w638] -> w581
            tunnel: w579 -> [w611 w637]
            tunnel: [w616 w636] -> w578
            tunnel: w574 -> [w609 _]
            tunnel: w573 -> [w610 _]
            frame False {
              # "position"
              # "area"
              n255 = case shown="True" w610 {
                tunnel: w615 -> [w631 w632]
                tunnel: w614 -> [w630 w633]
                tunnel: [w629 w635] -> w613
                tunnel: w609 -> [_ w634]
                frame False {
                  n256 = Add(x=w630, y=w631) -> (x+y=w628:i32)
                  n257 = Divide(x=w628, y=2 ("x")) -> (x/y=w626:dbl)
                  n258 = To Word Integer(number=w626) -> (16bit integer=w629:i16)
                }
                frame True {
                  n259 = call "compute_center_of_mass.vi"("end"=w632, "start"=w633, "array"=w634) -> ("center of  'mass'"=w635:u16)  [unwired: 8 in]
                }
              }
              n260 = Build Array (concatenate)(w611, w613) -> (w612:i32[])
              n261 = Build Array (concatenate)(w612, w617) -> (w616:i32[])
            }
            frame True {
              n262 = case shown="True" w657 {
                tunnel: w656 -> [w660 _]
                tunnel: w655 -> [w659 _]
                tunnel: w654 -> [w658 _]
                tunnel: w653 -> [_ w672]
                tunnel: w652 -> [_ w671]
                tunnel: w651 -> [_ w670]
                tunnel: w650 -> [w666 w675]
                tunnel: [w666 w672] -> w649
                tunnel: w648 -> [w665 w674]
                tunnel: [w665 w671] -> w647
                tunnel: w646 -> [w664 w673]
                tunnel: [w664 w670] -> w645
                tunnel: [w660 w675] -> w644
                tunnel: [w659 w674] -> w643
                tunnel: [w658 w673] -> w642
                tunnel: w641 -> [w662 _]
                tunnel: w640 -> [_ w669]
                tunnel: [TRUE w669] -> w639
                tunnel: [w662 TRUE] -> w638
                tunnel: w637 -> [w661 w667]
                tunnel: [w661 w667] -> w636
                frame False {
                  # "found last"
                }
                frame True {
                  # "found first"
                }
              }
            }
          }
        }
        n263 = And(x=w470, y=w469) -> (x .and. y?=w471:bool)
        n264 = case shown="True" w471 {
          tunnel: [w553 w572] -> w468
          tunnel: [w552 w572] -> w467
          tunnel: w470 -> [w553 _]
          tunnel: w469 -> [w552 _]
          tunnel: w465 -> [w550 w567]
          tunnel: w464 -> [w549 w563]
          tunnel: w463 -> [w548 w562]
          tunnel: w462 -> [w547 w568]
          tunnel: w461 -> [w546 w564]
          tunnel: w460 -> [w545 _]
          tunnel: w459 -> [w551 w566]
          tunnel: [w551 w570] -> w458
          tunnel: w457 -> [_ w560]
          tunnel: [w550 w558] -> w451
          tunnel: [w549 w558] -> w452
          tunnel: [w548 w558] -> w453
          tunnel: [w547 w558] -> w454
          tunnel: [w546 w558] -> w455
          tunnel: [w545 w558] -> w456
          frame False {
          }
          frame True {
            w558 = -1 ("x")
            w572 = FALSE
            # "area"
            # "pos"
            # "append first and last arrays"
            n265 = Subtract(x=w563, y=w562) -> (x-y=w565:i32)
            n266 = Add(x=w568, y=w567) -> (x+y=w569:i32)
            n267 = Add(x=w564, y=w565) -> (x+y=w556:i32)
            n268 = Divide(x=w556, y=2 ("x")) -> (x/y=w555:dbl)
            n269 = To Word Integer(number=w555) -> (16bit integer=w554:i16)
            n270 = Add(x=w554, y=w562) -> (x+y=w561:i32)
            n271 = call <vilib>:"quot_Remain.vi"("y"=w560, "x"=w561) -> ("x-y*floor(x/y)"=w559:i32)  [unwired: 1 out]
            n272 = Build Array (concatenate)(w566, w559) -> (w571:i32[])
            n273 = Build Array (concatenate)(w571, w569) -> (w570:i32[])
          }
        }
        n274 = case shown="True" w468 {
          tunnel: w467 -> [w530 w544]
          tunnel: [w530 w544] -> w466
          tunnel: w458 -> [w529 w535]
          tunnel: w456 -> [_ w538]
          tunnel: w455 -> [_ w539]
          tunnel: w454 -> [_ w536]
          tunnel: w453 -> [w526 w531]
          tunnel: w452 -> [w527 w532]
          tunnel: w451 -> [w528 w533]
          tunnel: [w529 w534] -> w450
          tunnel: [w528 w533] -> w447
          tunnel: [w527 w532] -> w448
          tunnel: [w526 w531] -> w449
          frame False {
          }
          frame True {
            # "area"
            # "pos"
            # "add first"
            n275 = Add(x=w538, y=w539) -> (x+y=w541:i32)
            n276 = Divide(x=w541, y=2 ("x")) -> (x/y=w543:dbl)
            n277 = To Word Integer(number=w543) -> (16bit integer=w537:i16)
            n278 = Build Array (concatenate)(w535, w537) -> (w540:i32[])
            n279 = Build Array (concatenate)(w540, w536) -> (w534:i32[])
          }
        }
        n280 = case shown="True" w466 {
          tunnel: w450 -> [w515 w521]
          tunnel: w449 -> [_ w520]
          tunnel: w448 -> [_ w519]
          tunnel: w447 -> [_ w518]
          tunnel: [w515 w516] -> w446
          frame False {
          }
          frame True {
            # "area"
            # "pos"
            # "add last"
            n281 = Add(x=w520, y=w519) -> (x+y=w525:i32)
            n282 = Divide(x=w525, y=2 ("x")) -> (x/y=w523:dbl)
            n283 = To Word Integer(number=w523) -> (16bit integer=w517:i16)
            n284 = Build Array (concatenate)(w521, w517) -> (w522:i32[])
            n285 = Build Array (concatenate)(w522, w518) -> (w516:i32[])
          }
        }
        "Array 2" <- w446
      }
    }
    n286 = Array Size(array=w30) -> (size(s)=w36:i32)
    n287 = Array Size(array=w57) -> (size(s)=w58:i32)
    n288 = case shown="True" w42 {
      tunnel: w79 -> [w758 w786]
      tunnel: w60 -> [w759 w784]
      tunnel: [w759 w779] -> w74
      tunnel: w80 -> [w757 w787]
      tunnel: [w758 w783] -> _
      tunnel: w36 -> [_ w778]
      tunnel: [w757 w777] -> w37
      frame False {
      }
      frame True {
        w764 = i16 0 items=["1", "2", "3", "4", "5", "6", "7", "8"] ("Line")
        w767 = i16 7 items=["1", "2", "3", "4", "5", "6", "7", "8"] ("Line")
        (unwired) i16 255 ("Start X")
        # "max value"
        n289 = stacked-sequence {
          tunnel: w787 -> [w836]
          tunnel: [w835] -> w777
          tunnel: w786 -> [w826]
          tunnel: w784 -> [w827]
          tunnel: [w827] -> w785
          tunnel: [w826] -> w783
          tunnel: w778 -> [w825]
          frame #0 {
            # "end"
            n290 = Array Size(array=w826) -> (size(s)=w830:i32)
            n291 = Divide(x=w830, y=3) -> (x/y=w828:dbl)
            n292 = for {
              N: w828 -> [_]
              shift-right: [w856] -> _
              shift-left: i16 0 ("Start X") -> [w853]
              shift-right: [w855] -> _
              shift-left: i16 1 ("Start X") -> [w852]
              shift-right: [w844] -> w834
              shift-left: i16[] [] -> [w846]
              tunnel: w826 -> [w851]
              shift-right: [w849] -> w832
              shift-left: i16 0 ("Start X") -> [w850]
              w857 = 3 ("y")
              # "end"
              # "start"
              n293 = Index Array(array=w851, index=w852) -> (element=w849:i32)
              n294 = Index Array(array=w851, index=w853) -> (element=w848:i32)
              n295 = Add(x=w853, y=w857) -> (x+y=w856:i32)
              n296 = Subtract(x=w849, y=w848) -> (x-y=w847:i32)
              n297 = Subtract(x=w848, y=w850) -> (x-y=w854:i32)
              n298 = Add(x=w852, y=w857) -> (x+y=w855:i32)
              n299 = for {
                N: w854 -> [_]
                shift-right: [w862] -> w845
                shift-left: w846 -> [w863]
                n300 = Build Array (concatenate)(w863, i16 0 ("Start X")) -> (w862:i16[])
              }
              n301 = for {
                N: w847 -> [_]
                shift-right: [w858] -> w844
                shift-left: w845 -> [w859]
                n302 = Build Array (concatenate)(w859, i16 1 ("Start X")) -> (w858:i16[])
              }
            }
            n303 = Subtract(x=w825, y=w832) -> (x-y=w831:i32)
            n304 = for {
              N: w831 -> [_]
              shift-right: [w842] -> w833
              shift-left: w834 -> [w843]
              n305 = Build Array (concatenate)(w843, i16 0 ("Start X")) -> (w842:i16[])
            }
            n306 = Multiply(x=w833, y=w836) -> (x*y=w835:i16[])
          }
        }
        n307 = for {
          tunnel: "array 4" -> [w793] mode=indexing
          tunnel: "array 4" -> [w795]
          tunnel: [w795] -> w772
          shift-right: [w792] -> w766
          shift-left: i16 -1 ("Start X") -> [w791]
          n308 = Greater?(x=w793, y=w791) -> (0:w794:bool)
          n309 = case shown="True" w794 {
            tunnel: w793 -> [_ w797]
            tunnel: [w796 w797] -> w792
            tunnel: w791 -> [w796 _]
            frame False {
            }
            frame True {
            }
          }
        }
        n310 = case shown="False" "clear (T/F) 3" {
          tunnel: "NXT 11" -> [w788 w790]
          tunnel: [w788 w789] -> w763
          frame False {
          }
          frame True {
            n311 = call-poly <vilib>:"PolyDisplay.vi"("NXT"=w790) -> ("NXT"=w789:T1)  [unwired: 3 in]
          }
        }
        n312 = Array Size(array=w772) -> (size(s)=w762:i32)
        n313 = Divide(x=i16 30 ("Start X"), y=w766) -> (x/y=w776:dbl)
        n314 = call-poly <vilib>:"PolyDisplay.vi"("number"=w762, "NXT"=w763, "Line"=w764) -> ("NXT"=w761:T1)  [unwired: 1 in]
        n315 = call-poly <vilib>:"PolyDisplay.vi"("number"=w766, "NXT"=w761, "Line"=w767) -> ("NXT"=w768:T1)  [unwired: 1 in]
        n316 = call-poly <vilib>:"PolyDisplay.vi"("Circle Parameters"=T2 {"Origin X"=49, "Origin Y"=31, "Radius"=30}, "NXT"=w768) -> ("NXT"=w769:T1)  [unwired: 2 in]
        n317 = for {
          N: w762 -> [_]
          tunnel: [w817] -> w774
          tunnel: w776 -> [w821]
          tunnel: w769 -> [w820]
          tunnel: w772 -> [w819]
          tunnel: w762 -> [w802]
          i -> [w803]
          w811 = i16 49 ("Start X")
          w809 = i16 31 ("Start X")
          # "shift"
          # "dx"
          # "dy"
          # "radians"
          # "magnitude"
          n318 = Index Array(array=w819, index=w803) -> (element=w818:i32)
          n319 = Divide(x=w803, y=w802) -> (x/y=w816:dbl)
          n320 = Multiply(x=w818, y=w821) -> (x*y=w810:dbl)
          n321 = Multiply(x=w816, y=6.283185307179586 ("Pi Multiplied By 2")) -> (x*y=w800:dbl)
          n322 = Add(x=w800, y=1.5707963267948966 ("Pi Divided By 2")) -> (x+y=w799:dbl)
          n323 = call <vilib>:"cosine.vi"("x"=w799) -> ("cos(x)"=w813:sgl)
          n324 = call <vilib>:"sine.vi"("x"=w799) -> ("sin(x)"=w814:sgl)
          n325 = Multiply(x=w813, y=w810) -> (x*y=w812:dbl)
          n326 = Multiply(x=w814, y=w810) -> (x*y=w801:dbl)
          n327 = Add(x=w812, y=w811) -> (x+y=w807:dbl)
          n328 = Add(x=w809, y=w801) -> (x+y=w805:dbl)
          n329 = To Word Integer(number=w807) -> (16bit integer=w806:i16)
          n330 = To Word Integer(number=w805) -> (16bit integer=w804:i16)
          n331 = Bundle("Start X"=w811, "Start X"=w809, w806, w804) -> (w808:cluster{"Start X":i16, "Start X":i16, i16, i16})  [unwired: 1 in]
          n332 = call-poly <vilib>:"PolyDisplay.vi"("Line Parameters"=w808, "NXT"=w820) -> ("NXT"=w817:T1)  [unwired: 2 in]
        }
        "NXT 12" <- w774
        n333 = call "radial_array_display.vi"("array"=w777, "NXT"=w785) -> ("NXT 2"=w782:T1)  [unwired: 9 in]
        n334 = while {
          tunnel: w782 -> [w823]
          tunnel: [w822] -> w780
          stop <- w824 stop-if-true
          n335 = call <vilib>:"readNXTButton.vi"("NXT"=w823) -> ("Yes/No"=w824:bool, "NXT"=w822:T1)  [unwired: 2 in]
        }
        n336 = call-poly <vilib>:"PolyWait.vi"("Time (1 sec)"=sgl 2.0, "NXT"=w780) -> ("NXT"=w779:T1)  [unwired: 2 in]
      }
    }
    n337 = Divide(x=w58, y=i16 2 ("Start X")) -> (x/y=w75:dbl)
    n338 = To Byte Integer(number=w75) -> (8bit integer=w73:i8)
    n339 = case shown="True" w42 {
      tunnel: w74 -> [w360 w371]
      tunnel: w57 -> [_ w365]
      tunnel: [w360 w361] -> w72
      frame False {
      }
      frame True {
        # "display list of areas"
        # "0 for list of positions"
        n340 = Array Size(array=w365) -> (size(s)=w369:i32)
        n341 = Divide(x=w369, y=2) -> (x/y=w367:dbl)
        n342 = To Word Integer(number=w367) -> (16bit integer=w366:i16)
        n343 = for {
          N: w366 -> [_]
          tunnel: w371 -> [w384]
          tunnel: [w384] -> w373
          shift-right: [w385] -> w372
          shift-left: "" ("Text") -> [w387]
          shift-right: [w382] -> _
          shift-left: i16 1 ("Start X") -> [w380]
          tunnel: w365 -> [w379]
          n344 = Index Array(array=w379, index=w380) -> (element=w378:i32)
          n345 = Add(x=w380, y=i16 2 ("Start X")) -> (x+y=w382:i16)
          n346 = call <vilib>:"NXT_floatToString.vi"("number"=w378) -> ("string"=w386:string)
          n347 = Concatenate Strings(w387, " " ("Text"), w386) -> (w385:string)
        }
        n348 = call-poly <vilib>:"PolyDisplay.vi"("Text"=w372, "NXT"=w373) -> ("NXT"=w364:T1)  [unwired: 2 in]
        n349 = while {
          tunnel: w364 -> [w376]
          tunnel: [w375] -> w362
          stop <- w377 stop-if-true
          n350 = call <vilib>:"readNXTButton.vi"("NXT"=w376) -> ("Yes/No"=w377:bool, "NXT"=w375:T1)  [unwired: 2 in]
        }
        n351 = call-poly <vilib>:"PolyWait.vi"("Time (1 sec)"=i16 1, "NXT"=w362) -> ("NXT"=w361:T1)  [unwired: 2 in]
      }
    }
    n352 = for {
      N: w73 -> [_]
      tunnel: w57 -> [w409]
      shift-right: [w408] -> _
      shift-left: i16 0 ("Start X") -> [w391]
      shift-right: [w407] -> _
      shift-left: i16 1 ("Start X") -> [w405]
      shift-right: [w400] -> w35
      shift-left: w69 -> [w395]
      shift-right: [w399] -> w68
      shift-left: w69 -> [w392]
      tunnel: w72 -> [w404]
      tunnel: i16 700 ("Start X") -> [w393]
      tunnel: [w404] -> w66
      tunnel: w36 -> [w389]
      w406 = i16 2 ("Start X")
      # "area"
      # "position"
      n353 = Less?(x=w392, y=w393) -> (x < y?=w402:bool)
      n354 = Index Array(array=w409, index=w405) -> (element=w401:i32)
      n355 = Index Array(array=w409, index=w391) -> (element=w394:i32)
      n356 = Divide(x=w389, y=i16 2 ("Start X")) -> (x/y=w388:dbl)
      n357 = Add(x=w405, y=w406) -> (x+y=w407:i16)
      n358 = Add(x=w391, y=w406) -> (x+y=w408:i16)
      n359 = Greater Or Equal?(x=w394, y=w388) -> (x >= y?=w397:bool)
      n360 = Greater Or Equal?(x=w395, y=w388) -> (x >= y?=w403:bool)
      n361 = case shown="True" w397 {
        tunnel: w394 -> [w410 w413]
        tunnel: [w410 w412] -> w396
        tunnel: w389 -> [_ w411]
        frame False {
        }
        frame True {
          n362 = Subtract(x=w411, y=w413) -> (x-y=w412:i32)
        }
      }
      n363 = case shown="True" w403 {
        tunnel: w395 -> [w439 w441]
        tunnel: [w439 w442] -> w398
        tunnel: w389 -> [_ w440]
        frame False {
        }
        frame True {
          n364 = Subtract(x=w440, y=w441) -> (x-y=w442:i32)
        }
      }
      n365 = case shown="True" w402 {
        tunnel: w394 -> [w422 w432]
        tunnel: w401 -> [w421 w430]
        tunnel: [w420 w431] -> w400
        tunnel: [w419 w429] -> w399
        tunnel: w398 -> [w416 _]
        tunnel: w396 -> [w415 _]
        tunnel: w395 -> [w418 w428]
        tunnel: w392 -> [w417 w427]
        tunnel: w392 -> [_ w434]
        frame False {
          n366 = Less?(x=w415, y=w416) -> (x < y?=w414:bool)
          n367 = case shown="False" w414 {
            tunnel: w422 -> [_ w426]
            tunnel: w421 -> [_ w425]
            tunnel: [w424 w426] -> w420
            tunnel: [w423 w425] -> w419
            tunnel: w418 -> [w424 _]
            tunnel: w417 -> [w423 _]
            frame False {
            }
            frame True {
            }
          }
        }
        frame True {
          n368 = Greater?(x=w430, y=w434) -> (0:w433:bool)
          n369 = case shown="True" w433 {
            tunnel: w432 -> [_ w438]
            tunnel: [w435 w438] -> w431
            tunnel: w430 -> [_ w437]
            tunnel: [w436 w437] -> w429
            tunnel: w428 -> [w435 _]
            tunnel: w427 -> [w436 _]
            frame False {
            }
            frame True {
            }
          }
        }
      }
    }
    n370 = Divide(x=w36, y=i16 2 ("Start X")) -> (x/y=w62:dbl)
    n371 = Greater Or Equal?(x=w35, y=w62) -> (x >= y?=w65:bool)
    n372 = Greater Or Equal?(x=w35, y=w62) -> (x >= y?=w28:bool)
    "right(T)/left(F)" <- w28
    n373 = Divide(x=w35, y=w36) -> (x/y=w34:dbl)
    n374 = case shown="True" w65 {
      tunnel: w35 -> [w270 w272]
      tunnel: [w270 w271] -> w64
      tunnel: w36 -> [_ w273]
      frame False {
      }
      frame True {
        n375 = Subtract(x=w273, y=w272) -> (x-y=w271:i32)
      }
    }
    n376 = Multiply(x=6.283185307179586 ("Pi Multiplied By 2"), y=w34) -> (x*y=w33:dbl)
    n377 = Add(x=1.5707963267948966 ("Pi Divided By 2"), y=w33) -> (x+y=w31:dbl)
    n378 = Divide(x=w64, y=w36) -> (x/y=w38:dbl)
    n379 = Multiply(x=i16 360 ("Start X"), y=w38) -> (x*y=w29:dbl)
    "angle" <- w29
    n380 = case shown="True" w42 {
      tunnel: w66 -> [w274 w293]
      tunnel: [w274 w317] -> w27
      tunnel: w68 -> [_ _]
      tunnel: w31 -> [_ w312]
      tunnel: w29 -> [_ w313]
      tunnel: w37 -> [_ w297]
      tunnel: w28 -> [_ w296]
      frame False {
        # "turn right"
      }
      frame True {
        w279 = i16 0 items=["1", "2", "3", "4", "5", "6", "7", "8"] ("Line")
        w282 = i16 7 items=["1", "2", "3", "4", "5", "6", "7", "8"] ("Line")
        (unwired) i16 255 ("Start X")
        w309 = i16 100 ("Start X")
        w314 = i16 2 items=["1", "2", "3", "4", "5", "6", "7", "8"] ("Line")
        w316 = i16 1 items=["1", "2", "3", "4", "5", "6", "7", "8"] ("Line")
        w306 = i16 49 ("Start X")
        w305 = i16 31 ("Start X")
        # "max value"
        # "dont erase"
        # "turn left"
        n381 = case shown="False" w296 {
          tunnel: ["L" "R"] -> w295
          frame False {
          }
          frame True {
          }
        }
        n382 = call-poly <vilib>:"PolyDisplay.vi"("NXT"=w293) -> ("NXT"=w292:T1)  [unwired: 3 in]
        n383 = for {
          tunnel: "array 5" -> [w326] mode=indexing
          tunnel: "array 5" -> [w328]
          tunnel: [w328] -> w287
          shift-right: [w325] -> w281
          shift-left: i16 -1 ("Start X") -> [w324]
          n384 = Greater?(x=w326, y=w324) -> (0:w327:bool)
          n385 = case shown="True" w327 {
            tunnel: w326 -> [_ w330]
            tunnel: [w329 w330] -> w325
            tunnel: w324 -> [w329 _]
            frame False {
            }
            frame True {
            }
          }
        }
        n386 = call <vilib>:"cosine.vi"("x"=w312) -> ("cos(x)"=w311:sgl)
        n387 = call <vilib>:"sine.vi"("x"=w312) -> ("sin(x)"=w310:sgl)
        n388 = call-poly <vilib>:"PolyDisplay.vi"("number"=w313, "NXT"=w292, "Line"=w316) -> ("NXT"=w320:T1)  [unwired: 1 in]
        n389 = Multiply(x=w309, y=w311) -> (x*y=w308:sgl)
        n390 = Multiply(x=w309, y=w310) -> (x*y=w307:sgl)
        n391 = call-poly <vilib>:"PolyDisplay.vi"("Text"=w295, "NXT"=w320, "Line"=w314) -> ("NXT"=w299:T1)  [unwired: 1 in]
        n392 = case shown="False" "clear (T/F) 4" {
          tunnel: "NXT 13" -> [w321 w323]
          tunnel: [w321 w322] -> w278
          frame False {
          }
          frame True {
            n393 = call-poly <vilib>:"PolyDisplay.vi"("NXT"=w323) -> ("NXT"=w322:T1)  [unwired: 3 in]
          }
        }
        n394 = Add(x=w306, y=w308) -> (x+y=w302:sgl)
        n395 = Add(x=w307, y=w305) -> (x+y=w301:sgl)
        n396 = To Word Integer(number=w302) -> (16bit integer=w304:i16)
        n397 = To Word Integer(number=w301) -> (16bit integer=w303:i16)
        n398 = Array Size(array=w287) -> (size(s)=w277:i32)
        n399 = call "radial_array_display.vi"("array"=w297, "clear (T/F)"=FALSE, "NXT"=w299) -> ("NXT 2"=w298:T1)  [unwired: 8 in]
        n400 = Bundle("Start X"=w306, "Start X"=w305, w304, w303) -> (w300:cluster{"Start X":i16, "Start X":i16, i16, i16})  [unwired: 1 in]
        n401 = Divide(x=i16 30 ("Start X"), y=w281) -> (x/y=w291:dbl)
        n402 = call-poly <vilib>:"PolyDisplay.vi"("Line Parameters"=w300, "NXT"=w298) -> ("NXT"=w315:T1)  [unwired: 2 in]
        n403 = while {
          tunnel: w315 -> [w358]
          tunnel: [w357] -> w318
          stop <- w359 stop-if-true
          n404 = call <vilib>:"readNXTButton.vi"("NXT"=w358) -> ("Yes/No"=w359:bool, "NXT"=w357:T1)  [unwired: 2 in]
        }
        n405 = call-poly <vilib>:"PolyDisplay.vi"("number"=w277, "NXT"=w278, "Line"=w279) -> ("NXT"=w276:T1)  [unwired: 1 in]
        n406 = call-poly <vilib>:"PolyDisplay.vi"("number"=w281, "NXT"=w276, "Line"=w282) -> ("NXT"=w283:T1)  [unwired: 1 in]
        n407 = call-poly <vilib>:"PolyDisplay.vi"("Circle Parameters"=T2 {"Origin X"=49, "Origin Y"=31, "Radius"=30}, "NXT"=w283) -> ("NXT"=w284:T1)  [unwired: 2 in]
        n408 = call-poly <vilib>:"PolyWait.vi"("Time (1 sec)"=i16 1, "NXT"=w318) -> ("NXT"=w317:T1)  [unwired: 2 in]
        n409 = for {
          N: w277 -> [_]
          tunnel: [w350] -> w289
          tunnel: w291 -> [w354]
          tunnel: w284 -> [w353]
          tunnel: w287 -> [w352]
          tunnel: w277 -> [w335]
          i -> [w336]
          w344 = i16 49 ("Start X")
          w342 = i16 31 ("Start X")
          # "shift"
          # "dx"
          # "dy"
          # "radians"
          # "magnitude"
          n410 = Index Array(array=w352, index=w336) -> (element=w351:i32)
          n411 = Divide(x=w336, y=w335) -> (x/y=w349:dbl)
          n412 = Multiply(x=w351, y=w354) -> (x*y=w343:dbl)
          n413 = Multiply(x=w349, y=6.283185307179586 ("Pi Multiplied By 2")) -> (x*y=w333:dbl)
          n414 = Add(x=w333, y=1.5707963267948966 ("Pi Divided By 2")) -> (x+y=w332:dbl)
          n415 = call <vilib>:"cosine.vi"("x"=w332) -> ("cos(x)"=w346:sgl)
          n416 = call <vilib>:"sine.vi"("x"=w332) -> ("sin(x)"=w347:sgl)
          n417 = Multiply(x=w346, y=w343) -> (x*y=w345:dbl)
          n418 = Multiply(x=w347, y=w343) -> (x*y=w334:dbl)
          n419 = Add(x=w345, y=w344) -> (x+y=w340:dbl)
          n420 = Add(x=w342, y=w334) -> (x+y=w338:dbl)
          n421 = To Word Integer(number=w340) -> (16bit integer=w339:i16)
          n422 = To Word Integer(number=w338) -> (16bit integer=w337:i16)
          n423 = Bundle("Start X"=w344, "Start X"=w342, w339, w337) -> (w341:cluster{"Start X":i16, "Start X":i16, i16, i16})  [unwired: 1 in]
          n424 = call-poly <vilib>:"PolyDisplay.vi"("Line Parameters"=w341, "NXT"=w353) -> ("NXT"=w350:T1)  [unwired: 2 in]
        }
        "NXT 14" <- w289
      }
    }
    "NXT 2" <- w27
    n425 = call <vilib>:"ResetMotor.vi"("NXT"=w27, "Port (All Ports)"=w91) -> ("NXT"=w90:T1)  [unwired: 2 in]
    n426 = call "rotate.vi"("degrees to  rotate"=w29, "right(T)/left(F)"=w28, "power"=u16 75, "NXT 2"=w90) -> ("NXT"=w89:T1)  [unwired: 7 in]
    n427 = call "drive_forward.vi"("min distance"=u16 30 ("power"), "power"=u16 60, "NXT"=w89) -> ("stuck"=w85:bool, "NXT 2"=w84:T1)  [unwired: 7 in]
    n428 = case shown="True" w85 {
      tunnel: w84 -> [w1086 w1091]
      tunnel: [w1086 w1088] -> _
      frame False {
      }
      frame True {
        w1087 = T3 5 items=["Port A"=0, "Port B"=1, "Port C"=2, "Ports A & B"=4, "Ports A & C"=5, "Ports B & C"=6, "All Ports"=3] ("Output Port (All Ports)")
        # "robot is stuck"
        n429 = call-poly <vilib>:"PolySound.vi"("NXT"=w1091) -> ("NXT"=w1090:T1)  [unwired: 3 in]
        n430 = call <vilib>:"MotorDistance.vi"("Angle of Rotation (360)"=90, "NXT"=w1090, "Output Port (All Ports)"=w1087) -> ("NXT"=w1088:T1)  [unwired: 1 in]
      }
    }
  }
